vi "CatchError.vi"(7 "source":string, 8 "error in (no error)":errorcluster, 10 "next action in":string, 11 "Qbus in":refnum<class "Qbus.lvclass">) -> (0 "error out":errorcluster, 2 "next action out":string, 3 "Qbus out":refnum<class "Qbus.lvclass">)   [LabVIEW 2017, in "Qbus.lvclass"]
uses:
  <vilib>/addons/Qbus/Qbus.lvclass
  <vilib>/addons/Qbus/Qbus.lvclass/Qbus.ctl
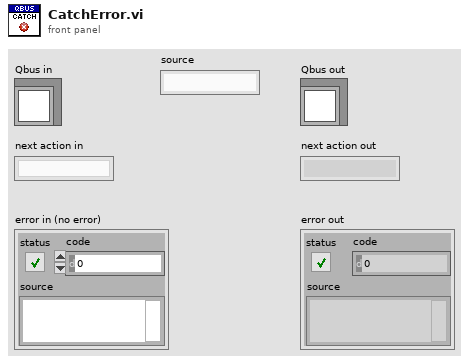
[diagram p1: front panel]
types:
  T1 = typedef "Qbus.lvclass/data.ctl" = cluster{"Queues":variant, "Subscriptions":variant, "MasterQ":string}
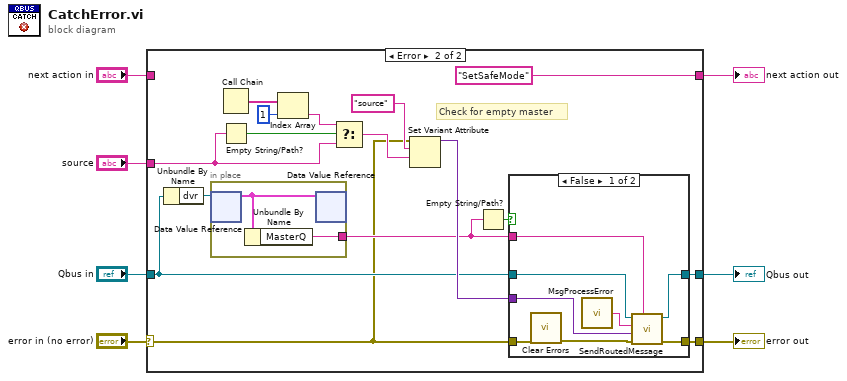
[diagram p0: block diagram]
diagram:
  n1 = case shown="Error" "error in (no error)" {
    selector: "error in (no error)" -> [w8 w11]
    tunnel: "source" -> [_ w21]
    tunnel: [w10 "SetSafeMode" ("NextAction")] -> w5
    tunnel: "next action in" -> [w10 _]
    tunnel: "Qbus in" -> [w9 w15]
    tunnel: [w9 w24] -> w2
    tunnel: [w8 w23] -> w1
    frame No Error {
    }
    frame Error {
      # "Check for empty master"
      n2 = Unbundle By Name(w15) -> ("dvr"=w14:refnum<data-value>)
      n3 = in-place {
        in-place-border: [w37] -> w13
        n4 = in-place-dvr #1(w14) -> (w38:T1)  [unwired: 1 out]
        n5 = Unbundle By Name(w38) -> ("MasterQ"=w37:string)
        n6 = in-place-dvr #1(w38) -> ()  [unwired: 2 out]
      }
      n7 = Call Chain() -> (call chain=w18:string[])
      n8 = Empty String/Path?(string/path=w21) -> (empty?=w19:bool)
      n9 = Index Array(array=w18, index=1) -> (element=w16:string)
      n10 = Select(t=w16, s=w19, f=w21) -> (s? t:f=w20:string)
      n11 = Set Variant Attribute(Variant=w11, name="source", value=w20) -> (Variant out=w22:variant)  [unwired: 1 in, 2 out]
      n12 = Empty String/Path?(string/path=w13) -> (empty?=w12:bool)
      n13 = case shown="False" w12 {
        tunnel: w11 -> [w28 w35]
        tunnel: [w34 w36] -> w24
        tunnel: [w33 w35] -> w23
        tunnel: w22 -> [w32 _]
        tunnel: w15 -> [w31 w36]
        tunnel: w13 -> [w29 _]
        frame False {
          n14 = call <vilib>:"Clear Errors.vi"("error in (no error)"=w28) -> ("error out"=w27:errorcluster)  [unwired: 5 in, 1 out]
          n15 = call <vilib>:"MsgProcessError.vi"() -> ("message name"=w30:string)  [unwired: 5 in]
          n16 = call <vilib>:"SendRoutedMessage.vi"("listener process"=w29, "error in (no error)"=w27, "message value"=w32, "message name"=w30, "Qbus in"=w31) -> ("error in (no error)"=w33:errorcluster, "Qbus out"=w34:refnum<class "Qbus.lvclass">)  [unwired: 5 in]
        }
        frame True {
        }
      }
    }
  }
  "error out" <- w1
  "next action out" <- w5
  "Qbus out" <- w2
